vi "Disable UI.vi"(8 "error in (no error)":errorcluster, 11 "Operator UI Actor in":refnum<class "Server UI.lvclass">) -> (0 "error out":errorcluster, 3 "Operator UI Actor out":refnum<class "Server UI.lvclass">)   [LabVIEW 2026, in "Server UI.lvlib" / "Server UI.lvclass"]
uses:
  Server UI.lvclass
  Server UI.lvclass/Server UI.ctl
  Read Start Server.vi
  framework/Msmt UI/Measurement UI.lvclass
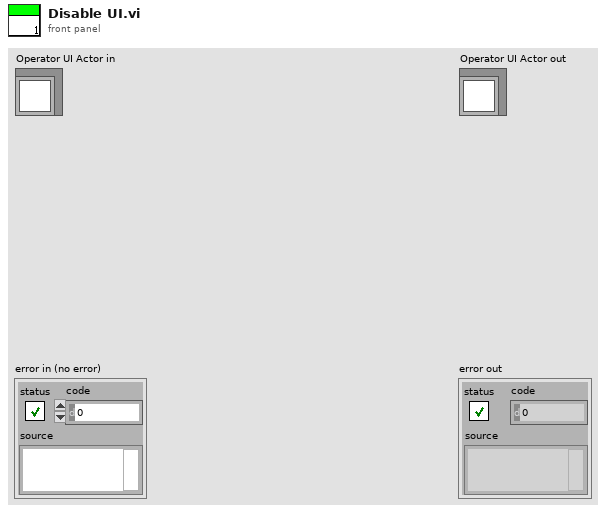
[diagram p1: front panel]
types:
  T1 = enum8{"Enabled", "Disabled", "Disabled and Grayed Out"}
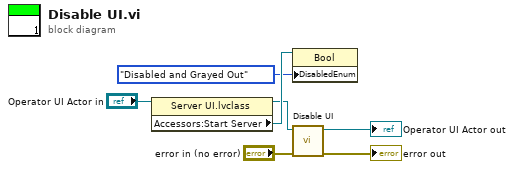
[diagram p0: block diagram]
diagram:
  n1 = property class="Server UI.lvclass"(reference="Operator UI Actor in") -> (reference out=w1:refnum<class "Server UI.lvclass">, "Accessors:Start Server"=w3:refnum<vi>)  [unwired: 1 in, 1 out]
  n2 = property class="Bool"(reference=w3, "DisabledEnum"=T1."Disabled and Grayed Out" ("Disabled")) -> ()  [unwired: 1 in, 2 out]
  n3 = call-parent "Disable UI.vi"("error in (no error)"="error in (no error)", "Operator UI Actor in"=w1) -> ("error out"=→"error out":errorcluster, "Operator UI Actor out"=→"Operator UI Actor out":refnum<class "Server UI.lvclass">)  [unwired: 8 in]
